vi "TDC_DAQV_CountingRate_rpc.vi"(7 "bytes to read":i32=1600, 9 "UDP Config":bool=TRUE, 10 "timeout":dbl=4500.0) -> (0 "error out":errorcluster, 1 "trigger_rate":dbl[](array[numeric])=[-1.0, 1000.0, 1000.0, -1.0, -1.0, -1.0, -1.0, -1.0, -1.0, -1.0, -1.0, -1.0, -1.0, -1.0, -1.0, -1.0, -1.0, -1.0, -1.0, -1.0, -1.0, -1.0, -1.0, -1.0, -1.0, -1.0, -1.0, -1.0, -1.0, -1.0, -1.0, -1.0, -1.0, -1.0, -1.0, -1.0, -1.0, -1.0, -1.0, -1.0, -1.0, -1.0, -1.0, -1.0, -1.0, -1.0, -1.0, -1.0, -1.0, -1.0, -1.0, -1.0, -1.0, -1.0, -1.0, -1.0, -1.0, -1.0, -1.0, -1.0, -1.0, -1.0, -1.0, -1.0, -1.0, -1.0, -1.0, -1.0, -1.0, -1.0, -1.0, -1.0, -1.0, -1.0, -1.0, -1.0, -1.0, -1.0, -1.0, -1.0, -1.0, -1.0, -1.0, -1.0, -1.0, -1.0, -1.0, -1.0, -1.0, -1.0, -1.0, -1.0, -1.0, -1.0, -1.0, -1.0, -1.0, -1.0, -1.0, -1.0], 2 "time":dbl=15.088012218475342, 3 "rate":dbl=946.1619379016261)   [LabVIEW 2017]
panel:
  out "channel":u64=2
  out "无符号字节数组":u8[](array[numeric])=[3, 232]
  out "Out 2":u8=3 format="%.0x"
  in  "Array":string[](array[string])=["192.168.10.35"]
  in  "Thresholds":dbl=-0.03
  in  "one key for threshold":bool=TRUE
  out "DAC":dbl=8094.0
  in  "SMA mode":bool
  in  "Thresholds (mV)":dbl[](array[numeric])=[580.0, 580.0, 580.0, 580.0, 600.0, 600.0, 600.0, 600.0, 580.0, 580.0, 600.0, 600.0, 600.0, 600.0, 600.0, 600.0, 580.0, 580.0, 600.0, 600.0, 600.0, 600.0, 600.0, 600.0, 580.0, 580.0, 600.0, 600.0, 600.0, 600.0, 600.0, 600.0, 600.0, 600.0, 600.0, 600.0, 600.0, 600.0, 600.0, 600.0, 600.0, 600.0, 600.0, 600.0, 600.0, 600.0, 600.0, 600.0, 600.0, 600.0, 600.0, 600.0, 600.0, 600.0, 600.0, 600.0, 600.0, 600.0, 600.0, 600.0, 600.0, 600.0, 600.0, 600.0]
  out "Out":u8=3 format="%.0x"
  in  "error in (no error)":errorcluster
  out "数值":dbl=2.0
  out "sent number 2":u64=1000 format="%x"
  out "data 9":string
  out "sent number":u64 format="%x"
  out "substring 2":string
  out "channel number":u64=16 format="%x"
  out "substring":string
  out "array":dbl[](array[numeric])=[-1.0, -1.0, -1.0, -1.0, -1.0, -1.0, -1.0, -1.0, -1.0, -1.0, -1.0, -1.0, -1.0, -1.0, -1.0, -1.0, -1.0, -1.0, -1.0, -1.0, -1.0, -1.0, -1.0, -1.0, -1.0, -1.0, -1.0, -1.0, -1.0, -1.0, -1.0, -1.0, -1.0, -1.0, -1.0, -1.0, -1.0, -1.0, -1.0, -1.0, -1.0, -1.0, -1.0, -1.0, -1.0, -1.0, -1.0, -1.0, -1.0, -1.0, -1.0, -1.0, -1.0, -1.0, -1.0, -1.0, -1.0, -1.0, -1.0, -1.0, -1.0, -1.0, -1.0, -1.0, -1.0, -1.0, -1.0, -1.0, -1.0, -1.0, -1.0, -1.0, -1.0, -1.0, -1.0, -1.0, -1.0, -1.0, -1.0, -1.0, -1.0, -1.0, -1.0, -1.0, -1.0, -1.0, -1.0, -1.0, -1.0, -1.0, -1.0, -1.0, -1.0, -1.0, -1.0, -1.0, -1.0, -1.0, -1.0, -1.0]
  out "trigger number":u64=1000 format="%x"
  out "data 8":string
  out "concatenated string":string
  out "number":u32=35
  in  "factor":i32=2
  in  "stop":bool
  in  "timeout (ms)":i32=8400
  # "5A00 0000 0000 03E8 FC38 000B 800F 3F7B"
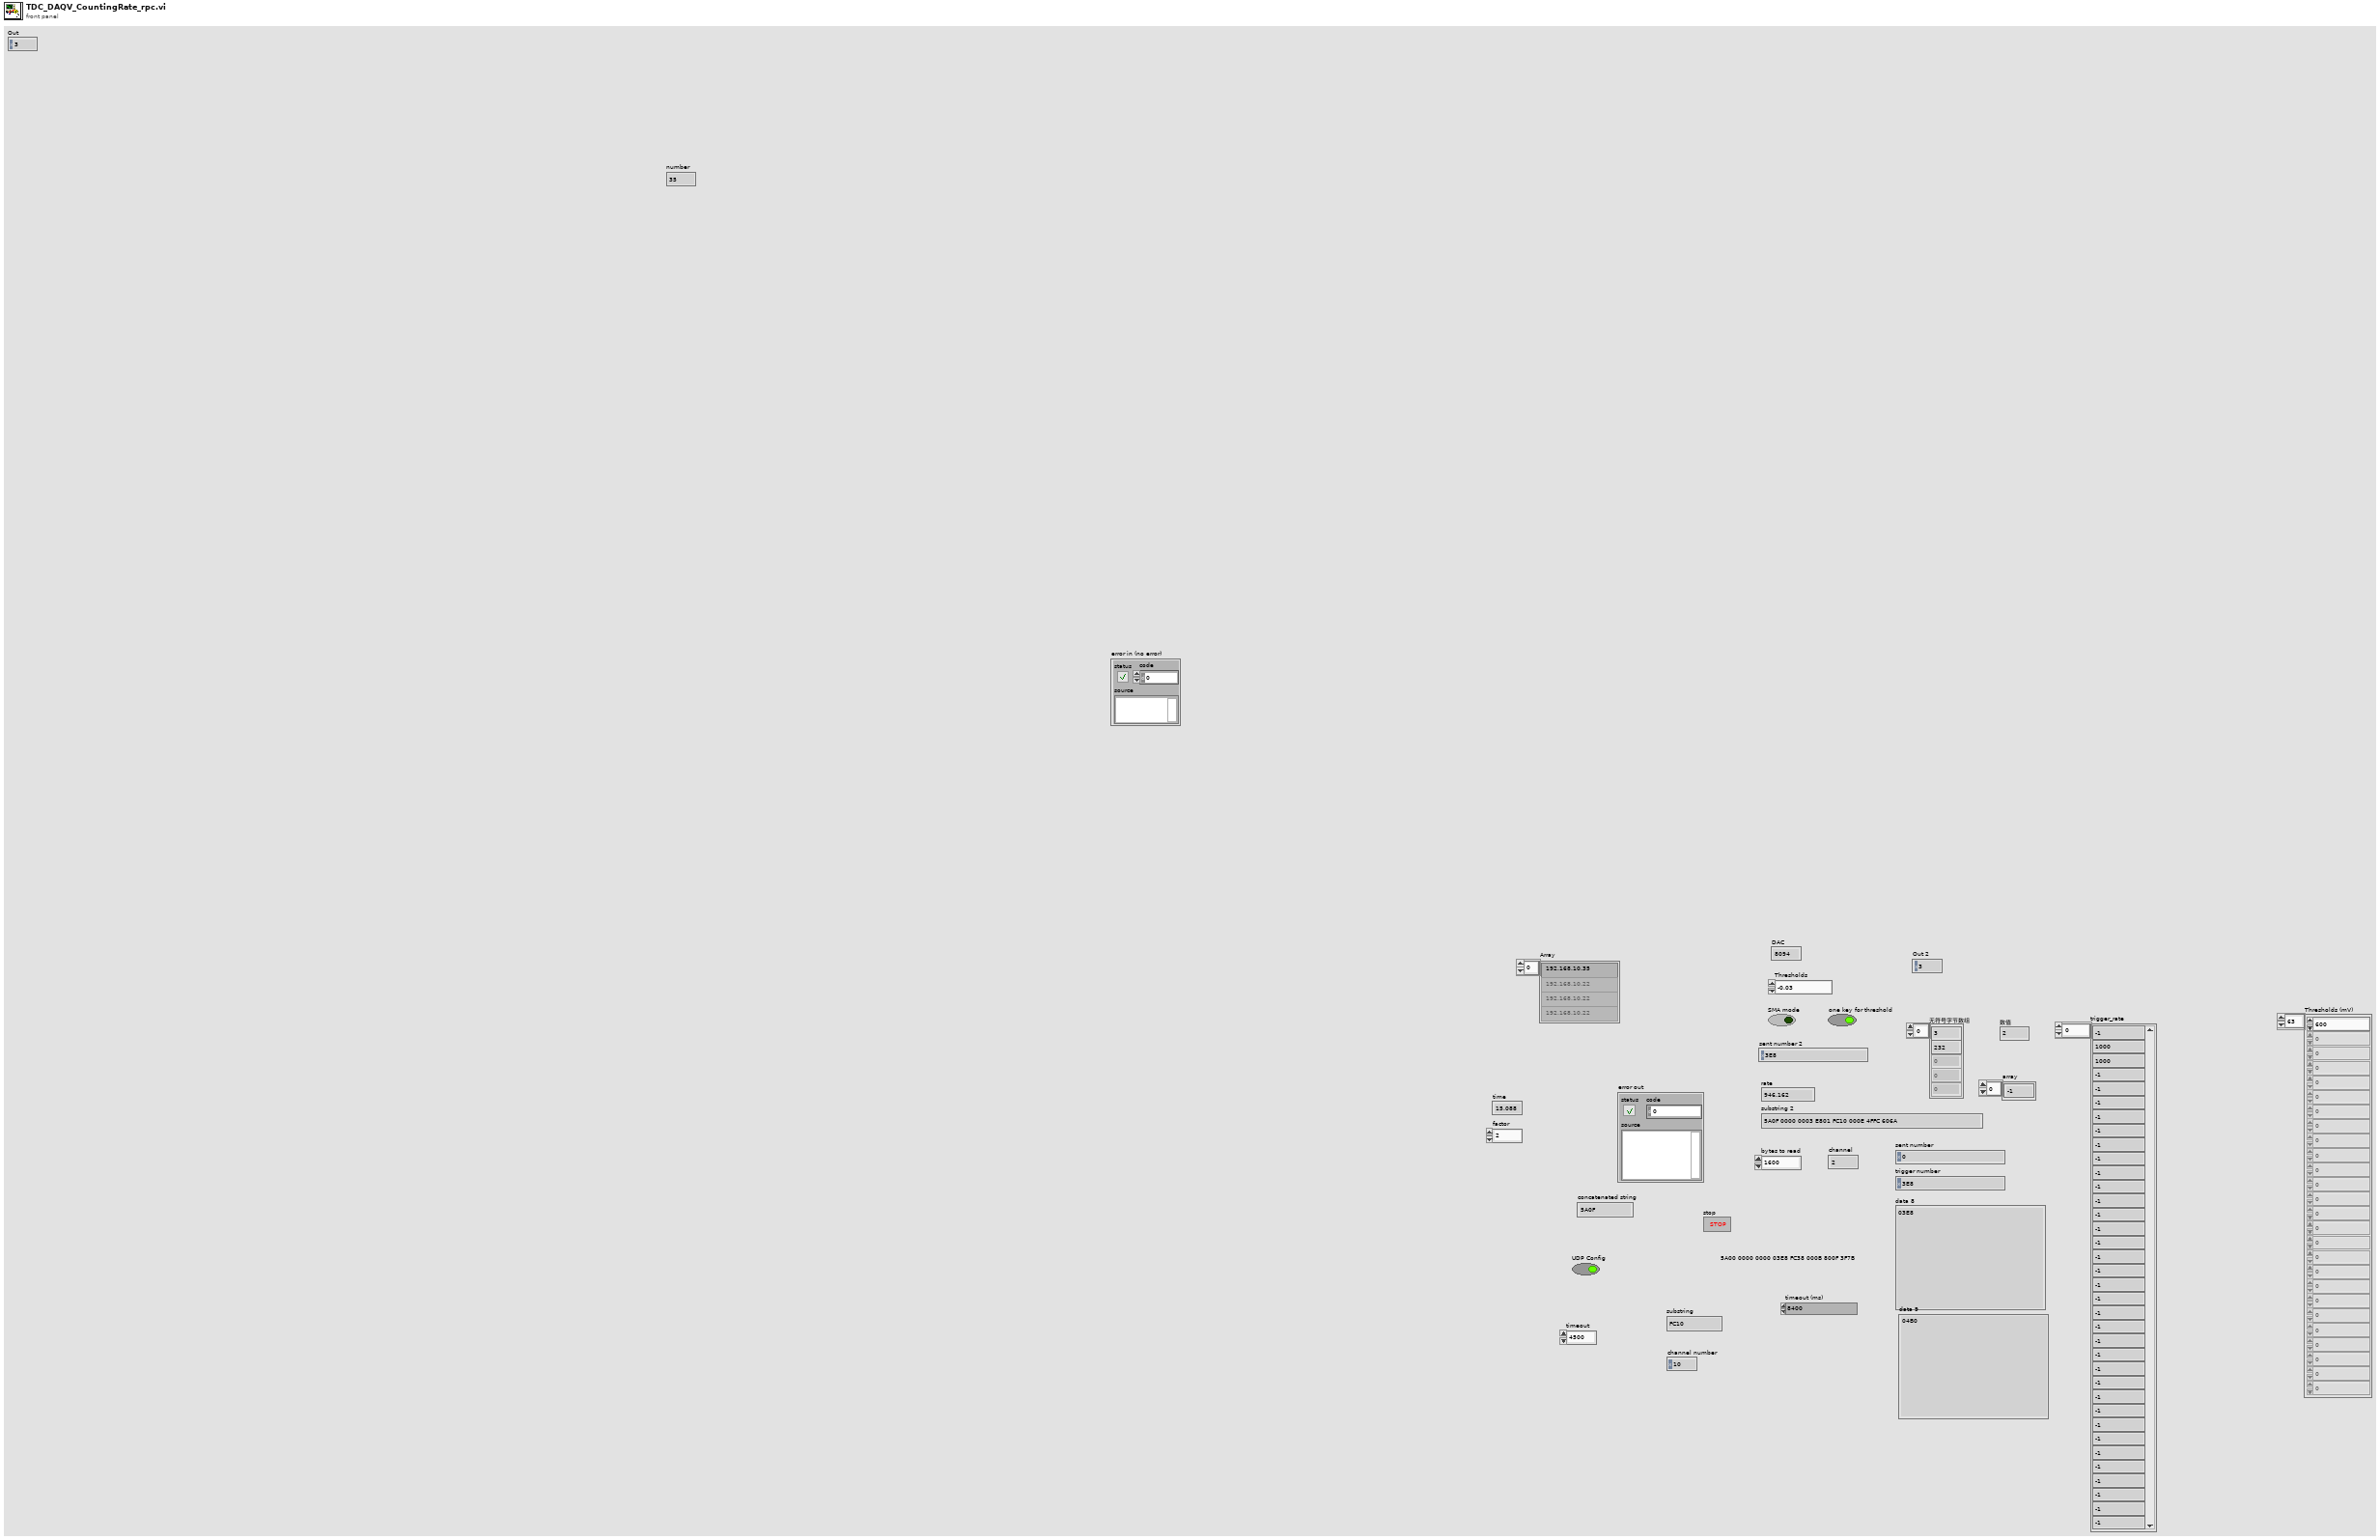
[diagram p1: front panel]
types:
  T1 = enum16{"Standard", "Buffered", "CRLF", "Immediate"}
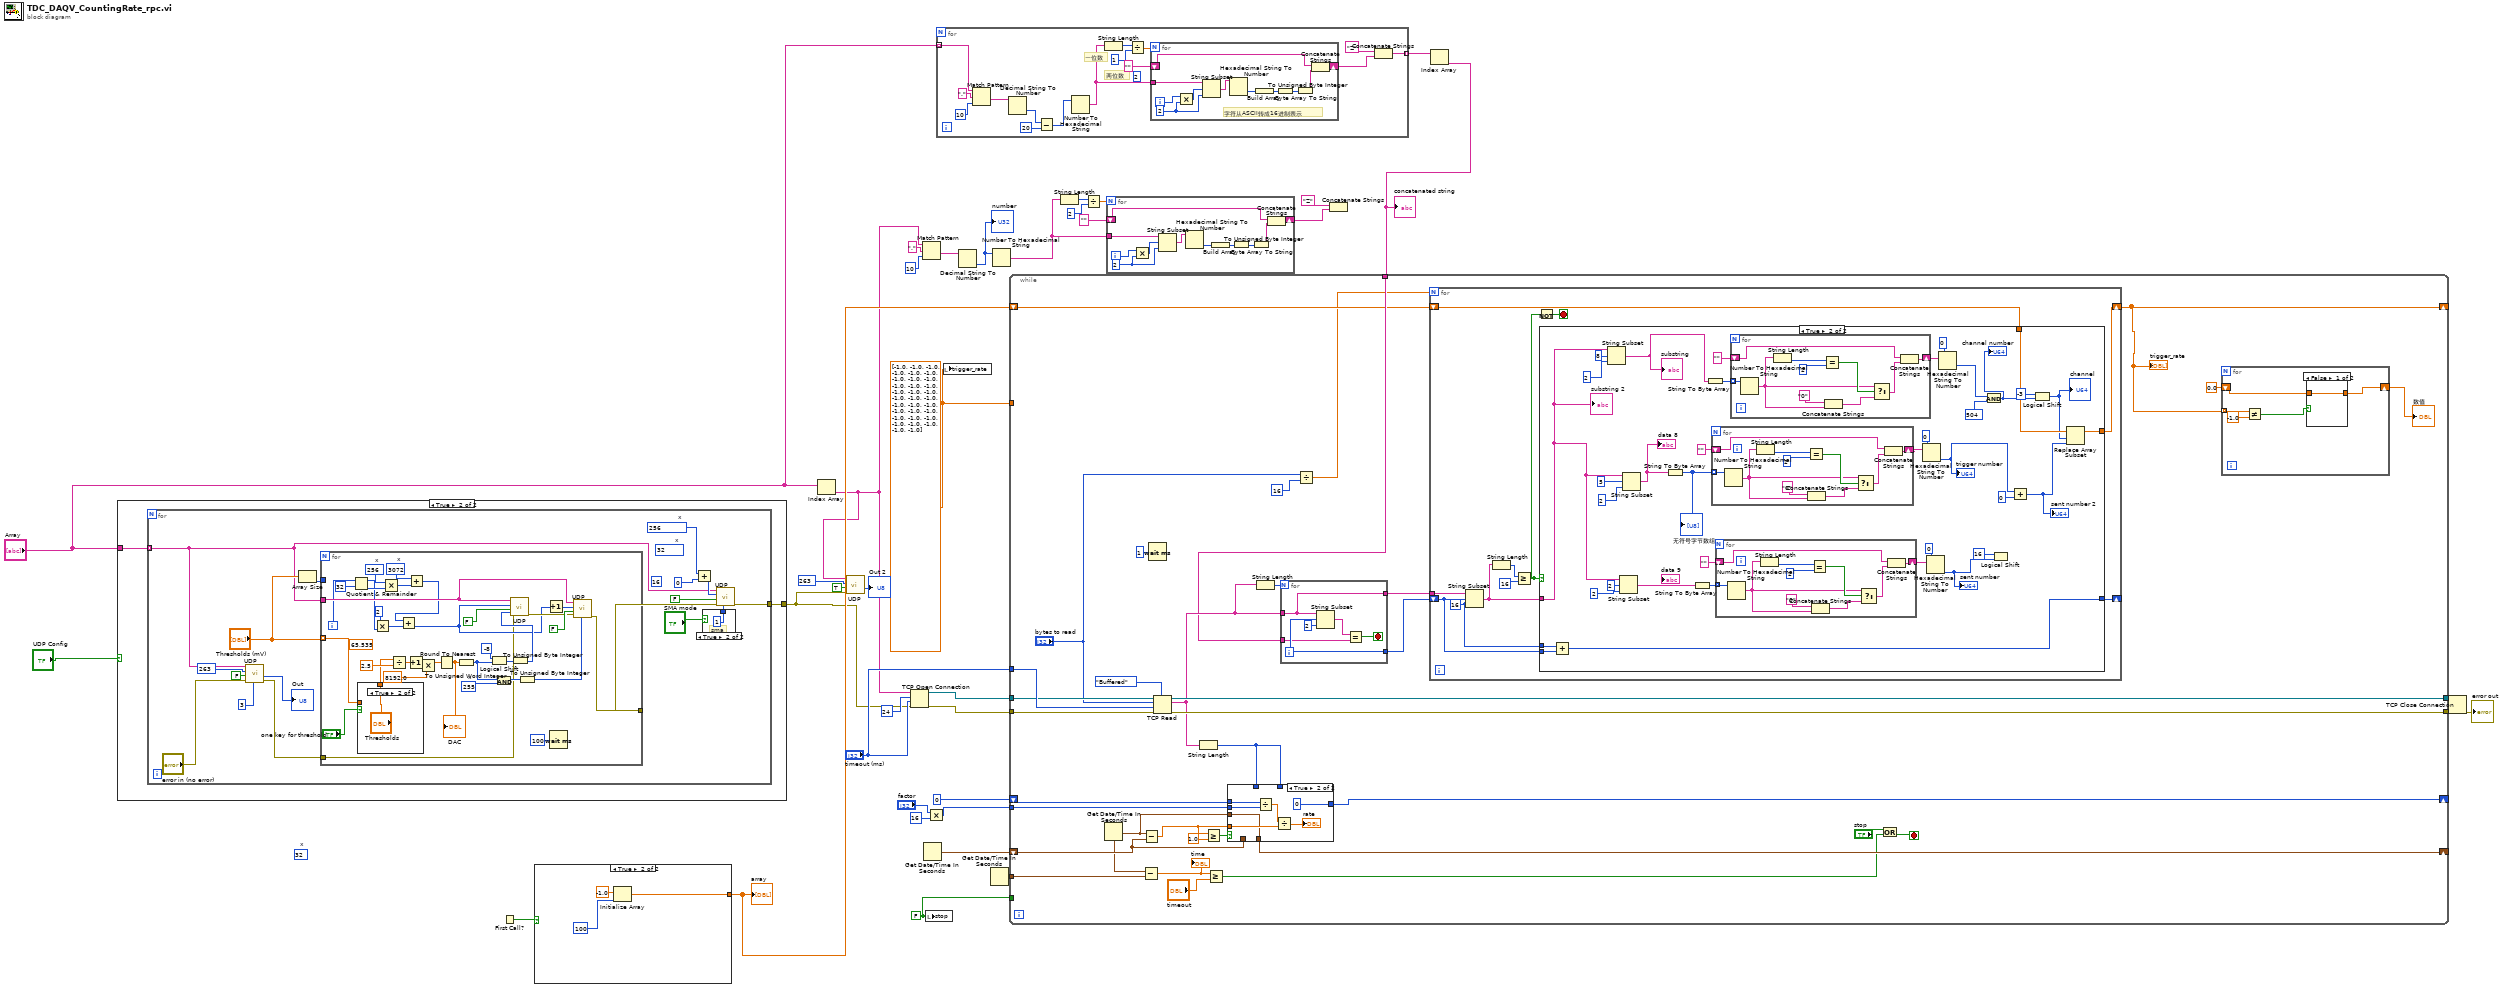
[diagram p0: block diagram]
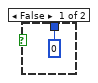
[diagram p3: hidden frame]
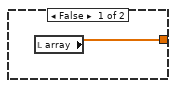
[diagram p5: hidden frame]
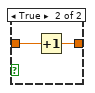
[diagram p6: hidden frame]
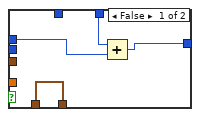
[diagram p8: hidden frame]
diagram:
  w10 = dbl[] [-1.0, -1.0, -1.0, -1.0, -1.0, -1.0, -1.0, -1.0, -1.0, -1.0, -1.0, -1.0, -1.0, -1.0, -1.0, -1.0, -1.0, -1.0, -1.0, -1.0, -1.0, -1.0, -1.0, -1.0, -1.0, -1.0, -1.0, -1.0, -1.0, -1.0, -1.0, -1.0] ("rate_array")
  w25 = FALSE ("stop")
  (unwired) u16 32  # x
  n1 = case shown="True" "UDP Config" {
    tunnel: "Array" -> [_ w38]
    tunnel: [_ w39] -> w3
    frame False {
    }
    frame True {
      n2 = for {
        tunnel: [w54] -> w39
        tunnel: w38 -> [w42] mode=indexing
        (unwired) u16 32  # x
        (unwired) u32 16 ("Address")
        w47 = u16 256  # x
        n3 = call "UDP.vi"("In"=u8 3, "error in (no error)"="error in (no error)", "Read (TRUE)"=FALSE, "Address"=u32 263, "IP address"=w42) -> ("error out"=w40:errorcluster, "Out"=→"Out":u8)  [unwired: 3 in, 1 out]
        n4 = Array Size(array="Thresholds (mV)") -> (size(s)=w51:i32)
        n5 = for {
          tunnel: w42 -> [w88]
          tunnel: "Thresholds (mV)" -> [w75] mode=indexing
          tunnel: [w78] -> w55
          tunnel: w51 -> [_]
          tunnel: w40 -> [w62]
          i -> [w70]
          (unwired) 65.535 ("y")
          w71 = u16 3072  # x
          w72 = u16 256  # x
          w84 = u16 255  # x
          n6 = Quotient & Remainder(x=w70, y=32) -> (x-y*floor(x/y)=w64:i32, floor(x/y)=w73:i32)
          n7 = case shown="True" "one key for threshold" {
            tunnel: [w94 "Thresholds"] -> w76
            tunnel: w75 -> [w94 _]
            frame False {
            }
            frame True {
            }
          }
          n8 = Multiply(x=2, y=w64) -> (x*y=w65:i32)
          n9 = Multiply(x=w72, y=w73) -> (x*y=w67:i32)
          n10 = Divide(x=w76, y=2.5) -> (x/y=w91:dbl)
          n11 = Increment(x=w91) -> (x+1=w61:dbl)
          n12 = Add(x=w71, y=w67) -> (x+y=w66:i32)
          n13 = Add(x=w66, y=w65) -> (x+y=w69:i32)
          n14 = Multiply(x=w61, y=8192.0) -> (x*y=w60:dbl)
          n15 = Round To Nearest(number=w60) -> (nearest integer value=w89:dbl)
          "DAC" <- w89
          n16 = To Unsigned Word Integer(number=w89) -> (unsigned 16bit integer=w80:u16)
          n17 = Logical Shift(y=i16 -8, x=w80) -> (x << y=w86:u16)
          n18 = And(x=w80, y=w84) -> (x .and. y?=w83:u16)
          n19 = To Unsigned Byte Integer(number=w86) -> (unsigned 8bit integer=w85:u8)
          n20 = call "UDP.vi"("In"=w85, "error in (no error)"=w62, "Read (TRUE)"=FALSE, "Address"=w69, "IP address"=w88) -> ("error out"=w79:errorcluster)  [unwired: 3 in, 2 out]
          n21 = To Unsigned Byte Integer(number=w83) -> (unsigned 8bit integer=w82:u8)
          n22 = Increment(x=w69) -> (x+1=w68:i32)
          n23 = Wait (ms)(milliseconds to wait=u32 100) -> ()  [unwired: 1 out]
          n24 = call "UDP.vi"("In"=w82, "error in (no error)"=w79, "Read (TRUE)"=FALSE, "Address"=w68, "IP address"=w88) -> ("error out"=w78:errorcluster)  [unwired: 3 in, 2 out]
        }
        n25 = Add(x=w47, y=u32 0 ("Address")) -> (x+y=w48:u32)
        n26 = case shown="True" "SMA mode" {
          tunnel: [u8 0 ("In") u8 1 ("In")] -> w53
          frame False {
          }
          frame True {
            # "sma"
          }
        }
        n27 = call "UDP.vi"("In"=w53, "error in (no error)"=w55, "Read (TRUE)"=FALSE, "Address"=w48, "IP address"=w42) -> ("error out"=w54:errorcluster)  [unwired: 3 in, 2 out]
      }
    }
  }
  n28 = First Call?() -> (First Call?: T/F=w12:bool)
  n29 = case shown="True" w12 {
    tunnel: [w96 w97] -> w11
    frame False {
      n30 = local read "array"() -> (w96:dbl[])
    }
    frame True {
      n31 = Initialize Array(-1.0 ("element"), 100 ("dimension size")) -> (w97:dbl[])
    }
  }
  "array" <- w11
  n32 = Index Array(array="Array") -> (element=w2:string)  [unwired: 1 in]
  n33 = call "UDP.vi"("error in (no error)"=w3, "Read (TRUE)"=TRUE, "Address"=u32 263, "IP address"=w2) -> ("Out"=→"Out 2":u8)  [unwired: 4 in, 2 out]
  n34 = TCP Open Connection(address=w2, remote port or service name=u16 24 ("port"), timeout ms (60000)="timeout (ms)", error in (no error)=w3) -> (connection ID=w35:refnum<k5>, error out=w36:errorcluster)  [unwired: 1 in]
  n35 = Match Pattern(string=w2, regular expression="." ("search string"), offset (0)=10) -> (after substring=w16:string)  [unwired: 3 out]
  n36 = Get Date/Time In Seconds() -> (seconds since 1Jan1904=w31:timestamp)
  n37 = local write "stop"(w25) -> ()
  n38 = Multiply(x="factor", y=16) -> (x*y=w27:i32)
  n39 = for {
    tunnel: [w101] -> w7 mode=indexing
    tunnel: "Array" -> [w100] mode=indexing
    (unwired) 2 ("y")
    # "一位数"
    # "两位数"
    n40 = Match Pattern(string=w100, regular expression="." ("search string"), offset (0)=10) -> (after substring=w107:string)  [unwired: 3 out]
    n41 = Decimal String To Number(string=w107) -> (number=w104:i32)  [unwired: 2 in, 1 out]
    n42 = Subtract(x=w104, y=20) -> (x-y=w103:i32)
    n43 = Number To Hexadecimal String(2:w103) -> (0:w106:string)  [unwired: 1 in]
    n44 = String Length(string=w106) -> (length=w112:i32)
    n45 = Divide(x=w112, y=1) -> (x/y=w113:dbl)
    n46 = for {
      N: w113 -> [_]
      shift-right: [w125] -> w102
      shift-left: "" ("format string") -> [w124]
      tunnel: w106 -> [w115]
      i -> [w123]
      w117 = 2 ("y")
      # "字符从ASCII转成16进制表示"
      n47 = Multiply(x=w123, y=w117) -> (x*y=w116:i32)
      n48 = String Subset(string=w115, offset (0)=w116, length (rest)=w117) -> (substring=w118:string)
      n49 = Hexadecimal String To Number(string=w118) -> (number=w122:u32)  [unwired: 2 in, 1 out]
      n50 = Build Array(w122) -> (w121:u32[])
      n51 = To Unsigned Byte Integer(number=w121) -> (unsigned 8bit integer=w120:u8[])
      n52 = Byte Array To String(unsigned byte array=w120) -> (string=w119:string)
      n53 = Concatenate Strings(w124, w119) -> (w125:string)
    }
    n54 = Concatenate Strings("Z", w102) -> (w101:string)
  }
  n55 = local write "trigger_rate"(w10) -> ()
  n56 = Decimal String To Number(string=w16) -> (number=w15:i32)  [unwired: 2 in, 1 out]
  "number" <- w15
  n57 = Get Date/Time In Seconds() -> (seconds since 1Jan1904=w24:timestamp)
  n58 = Number To Hexadecimal String(2:w15) -> (0:w14:string)  [unwired: 1 in]
  n59 = String Length(string=w14) -> (length=w21:i32)
  n60 = Divide(x=w21, y=2) -> (x/y=w22:dbl)
  n61 = for {
    N: w22 -> [_]
    shift-right: [w136] -> w13
    shift-left: "" ("format string") -> [w135]
    tunnel: w14 -> [w126]
    i -> [w134]
    w128 = 2 ("y")
    n62 = Multiply(x=w134, y=w128) -> (x*y=w127:i32)
    n63 = String Subset(string=w126, offset (0)=w127, length (rest)=w128) -> (substring=w129:string)
    n64 = Hexadecimal String To Number(string=w129) -> (number=w133:u32)  [unwired: 2 in, 1 out]
    n65 = Build Array(w133) -> (w132:u32[])
    n66 = To Unsigned Byte Integer(number=w132) -> (unsigned 8bit integer=w131:u8[])
    n67 = Byte Array To String(unsigned byte array=w131) -> (string=w130:string)
    n68 = Concatenate Strings(w135, w130) -> (w136:string)
  }
  n69 = Concatenate Strings("Z", w13) -> ()  [unwired: 1 out]
  n70 = Index Array(array=w7) -> (element=w6:string)  [unwired: 1 in]
  "concatenated string" <- w6
  n71 = while {
    tunnel: w36 -> [w171]
    tunnel: "timeout (ms)" -> [w170]
    tunnel: w35 -> [w169]
    tunnel: [w168] -> w34
    tunnel: [w167] -> w33
    shift-right: [w160] -> _
    shift-left: w31 -> [w164]
    shift-right: [w163] -> _
    shift-left: u32 0 ("milliseconds to wait") -> [w158]
    tunnel: w27 -> [w157]
    tunnel: w25 -> [_]
    tunnel: w24 -> [w151]
    tunnel: w6 -> [w145]
    shift-right: [w137] -> _
    shift-left: w11 -> [w144]
    tunnel: w10 -> [_]
    stop <- w154 stop-if-true
    n72 = Get Date/Time In Seconds() -> (seconds since 1Jan1904=w150:timestamp)
    n73 = Subtract(x=w150, y=w151) -> (x-y=w149:dbl)
    "time" <- w149
    n74 = Subtract(x=w150, y=w164) -> (x-y=w156:dbl)
    n75 = Wait (ms)(milliseconds to wait=u32 1) -> ()  [unwired: 1 out]
    n76 = TCP Read(connection ID=w169, bytes to read="bytes to read", error in (no error)=w171, 7:T1."Buffered" ("mode (standard)"), 9:w170) -> (connection ID out=w168:refnum<k5>, data out=w146:string, error out=w167:errorcluster)
    n77 = String Length(string=w146) -> (length=w159:i32)
    n78 = Greater Or Equal?(x=w156, y=1.0) -> (x >= y?=w162:bool)
    n79 = Greater Or Equal?(x=w149, y="timeout") -> (x >= y?=w152:bool)
    n80 = case shown="True" w162 {
      tunnel: w156 -> [_ w276]
      tunnel: w150 -> [_ w274]
      tunnel: [w269 w274] -> w160
      tunnel: w164 -> [w269 _]
      tunnel: w159 -> [_ _]
      tunnel: w159 -> [w268 _]
      tunnel: [w267 0] -> w163
      tunnel: w157 -> [_ w271]
      tunnel: w158 -> [w266 w270]
      frame False {
        n81 = Add(x=w268, y=w266) -> (x+y=w267:u32)
      }
      frame True {
        n82 = Divide(x=w270, y=w271) -> (x/y=w273:dbl)
        n83 = Divide(x=w273, y=w276) -> (x/y=→"rate":dbl)
      }
    }
    n84 = String Length(string=w146) -> (length=w148:i32)
    n85 = for {
      N: w148 -> [_]
      tunnel: w146 -> [w262]
      tunnel: [w262] -> w147
      tunnel: [w261] -> w143
      tunnel: w145 -> [w260]
      i -> [w261]
      stop <- w263 stop-if-true
      n86 = String Subset(string=w262, offset (0)=w261, length (rest)=2 ("length (rest)")) -> (substring=w264:string)
      n87 = Equal?(x=w264, y=w260) -> (x = y?=w263:bool)
    }
    n88 = Divide(x="bytes to read", y=16 ("length (rest)")) -> (x/y=w140:dbl)
    n89 = for {
      N: w140 -> [_]
      tunnel: w147 -> [w190]
      shift-right: [w188] -> w137
      shift-left: w144 -> [w189]
      shift-right: [w180] -> _
      shift-left: w143 -> [w181]
      stop <- w183 stop-if-true
      w182 = 16 ("length (rest)")
      n90 = String Subset(string=w190, offset (0)=w181, length (rest)=w182) -> (substring=w187:string)
      n91 = String Length(string=w187) -> (length=w186:i32)
      n92 = Greater Or Equal?(x=w186, y=16 ("length (rest)")) -> (x >= y?=w184:bool)
      n93 = Not(x=w184) -> (.not. x?=w183:bool)
      n94 = case shown="True" w184 {
        tunnel: w187 -> [_ w211]
        tunnel: w189 -> [w192 w210]
        tunnel: [w192 w209] -> w188
        tunnel: w181 -> [w191 w208]
        tunnel: w182 -> [_ w207]
        tunnel: [w191 w206] -> w180
        frame False {
        }
        frame True {
          n95 = Add(x=w207, y=w208) -> (x+y=w206:i32)
          n96 = String Subset(string=w211, offset (0)=8, length (rest)=2 ("length (rest)")) -> (substring=w214:string)
          "substring" <- w214
          n97 = String Subset(string=w211, offset (0)=2, length (rest)=2 ("length (rest)")) -> (substring=w201:string)
          n98 = String Subset(string=w211, offset (0)=5, length (rest)=2 ("length (rest)")) -> (substring=w221:string)
          "data 8" <- w221
          n99 = String To Byte Array(string=w221) -> (unsigned byte array=w223:u8[])
          "无符号字节数组" <- w223
          n100 = String To Byte Array(string=w201) -> (unsigned byte array=w204:u8[])
          n101 = String To Byte Array(string=w214) -> (unsigned byte array=w217:u8[])
          n102 = for {
            shift-right: [w258] -> w224
            shift-left: "" ("format string") -> [w255]
            tunnel: w223 -> [w259] mode=indexing
            n103 = Number To Hexadecimal String(2:w259) -> (0:w251:string)  [unwired: 1 in]
            n104 = String Length(string=w251) -> (length=w257:i32)
            n105 = Equal?(x=w257, y=2) -> (x = y?=w254:bool)
            n106 = Concatenate Strings("0" ("format string"), w251) -> (w253:string)
            n107 = Select(t=w251, s=w254, f=w253) -> (s? t:f=w250:string)
            n108 = Concatenate Strings(w255, w250) -> (w258:string)
          }
          n109 = for {
            shift-right: [w238] -> w203
            shift-left: "" ("format string") -> [w235]
            tunnel: w204 -> [w239] mode=indexing
            n110 = Number To Hexadecimal String(2:w239) -> (0:w231:string)  [unwired: 1 in]
            n111 = String Length(string=w231) -> (length=w237:i32)
            n112 = Equal?(x=w237, y=2) -> (x = y?=w234:bool)
            n113 = Concatenate Strings("0" ("format string"), w231) -> (w233:string)
            n114 = Select(t=w231, s=w234, f=w233) -> (s? t:f=w230:string)
            n115 = Concatenate Strings(w235, w230) -> (w238:string)
          }
          n116 = for {
            shift-right: [w248] -> w216
            shift-left: "" ("format string") -> [w245]
            tunnel: w217 -> [w249] mode=indexing
            n117 = Number To Hexadecimal String(2:w249) -> (0:w241:string)  [unwired: 1 in]
            n118 = String Length(string=w241) -> (length=w247:i32)
            n119 = Equal?(x=w247, y=2) -> (x = y?=w244:bool)
            n120 = Concatenate Strings("0" ("format string"), w241) -> (w243:string)
            n121 = Select(t=w241, s=w244, f=w243) -> (s? t:f=w240:string)
            n122 = Concatenate Strings(w245, w240) -> (w248:string)
          }
          n123 = Hexadecimal String To Number(string=w224, default (0uL)=u64 0 ("default (0 U32)")) -> (number=w198:u64)  [unwired: 1 in, 1 out]
          "trigger number" <- w198
          n124 = Hexadecimal String To Number(string=w203, default (0uL)=u64 0 ("default (0 U32)")) -> (number=w200:u64)  [unwired: 1 in, 1 out]
          "sent number" <- w200
          n125 = Hexadecimal String To Number(string=w216, default (0uL)=u64 0 ("default (0 U32)")) -> (number=w213:u64)  [unwired: 1 in, 1 out]
          n126 = And(x=w213, y=u64 504 ("default (0 U32)")) -> (x .and. y?=w194:u64)
          "channel number" <- w194
          n127 = Logical Shift(y=i16 16, x=w200) -> ()  [unwired: 1 out]
          n128 = Add(x=w198, y=u64 0) -> (x+y=w197:u64)
          "sent number 2" <- w197
          n129 = Logical Shift(y=i16 -3, x=w194) -> (x << y=w193:u64)
          "channel" <- w193
          n130 = Replace Array Subset(array=w210, new element=w197, index=w193) -> (w209:dbl[])
          "substring 2" <- w211
        }
      }
    }
    "trigger_rate" <- w137
    n131 = Or(x="stop", y=w152) -> (x .or. y?=w154:bool)
    n132 = for {
      tunnel: w137 -> [w176] mode=indexing
      shift-right: [w172] -> w138
      shift-left: 0.0 -> [w173]
      n133 = Not Equal?(x=w176, y=-1.0) -> (x != y?=w174:bool)
      n134 = case shown="False" w174 {
        tunnel: w173 -> [w177 w179]
        tunnel: [w177 w178] -> w172
        frame False {
        }
        frame True {
          n135 = Increment(x=w179) -> (x+1=w178:dbl)
        }
      }
    }
    "数值" <- w138
  }
  n136 = TCP Close Connection(connection ID=w34, error in (no error)=w33) -> (error out=→"error out":errorcluster)  [unwired: 1 in, 1 out]
